vi "Manual_Cam.vi"(4 "Frames in sequence":u32, 6 "Image in":variant, 7 "Camera-specific in":variant, 8 "Save path":path, 9 "Capture mode":enum16{"Single frame", "Sequence"}(ring), 10 "Exposure time (s)":dbl, 11 "Operation":T2(ring)) -> (3 "Status":T1, 5 "Camera-specific out":variant)   [LabVIEW 2015]
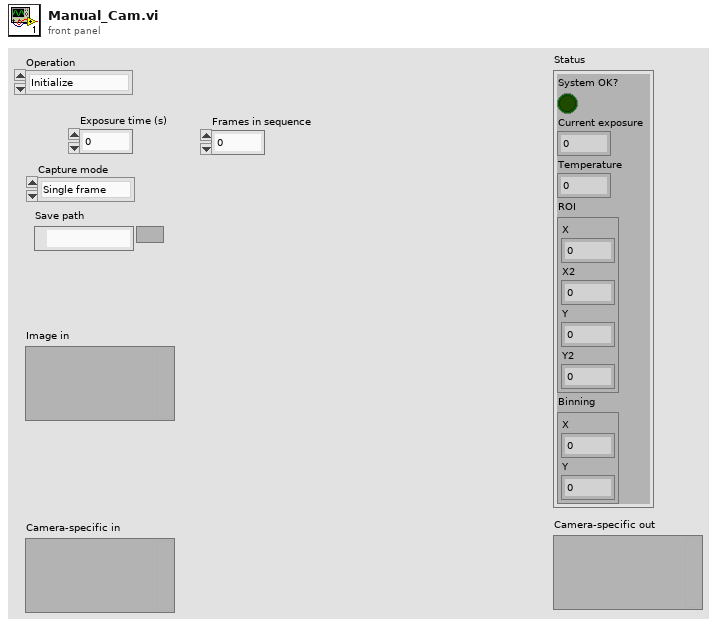
[diagram p1: front panel]
types:
  T1 = cluster{"System OK?":bool, "Current exposure":dbl, "Temperature":dbl, "ROI":cluster{"X":u32, "X2":u32, "Y":u32, "Y2":u32}, "Binning":cluster{"X":u32, "Y":u32}}
  T2 = enum16{"Initialize", "Shut down", "Set capture mode", "Set exposure", "Trigger and read", "Get status", "Other settings"}
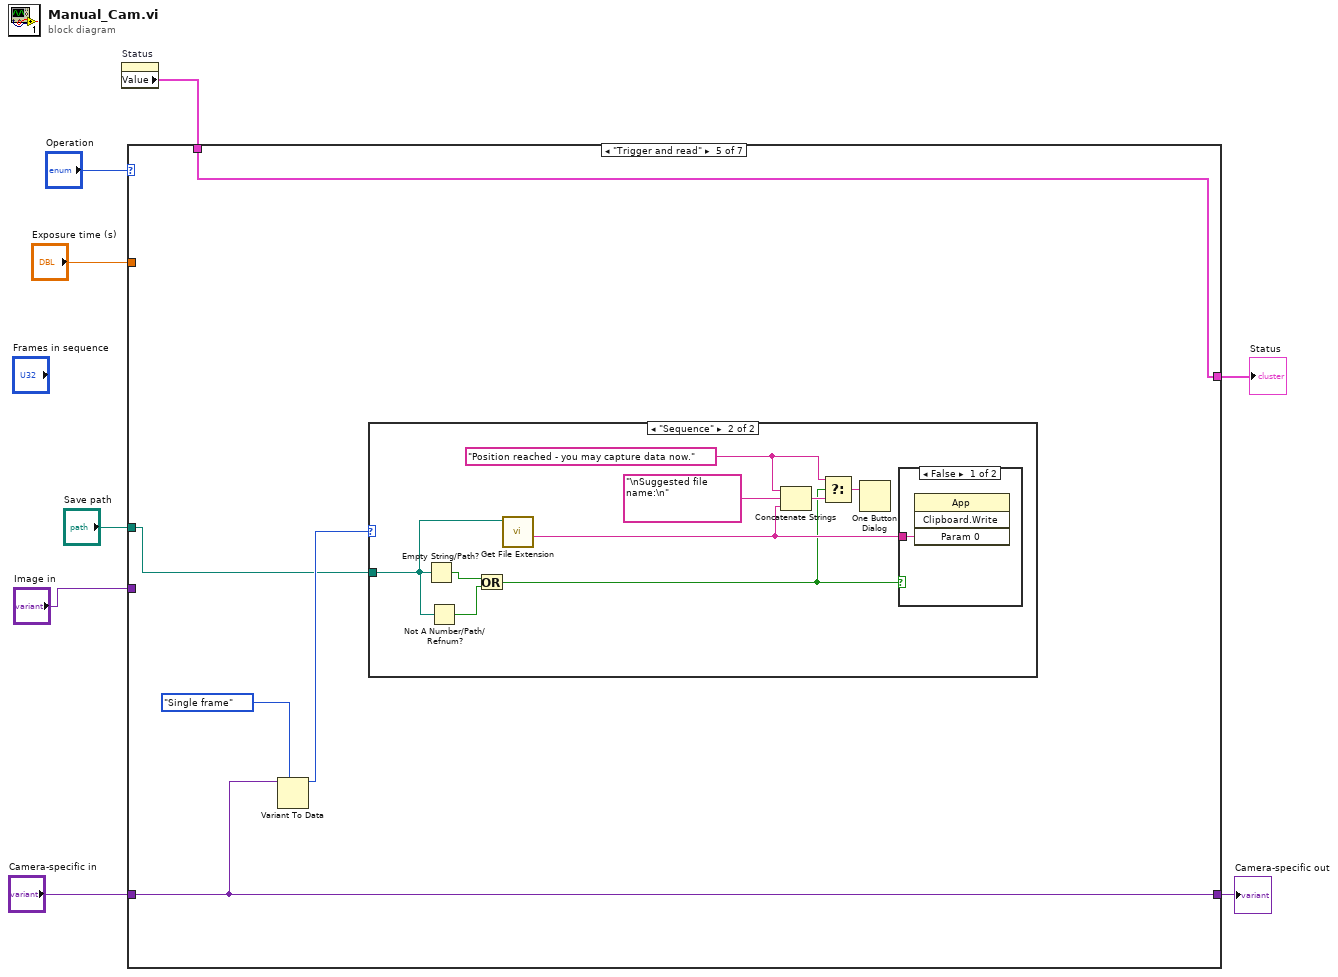
[diagram p0: block diagram]
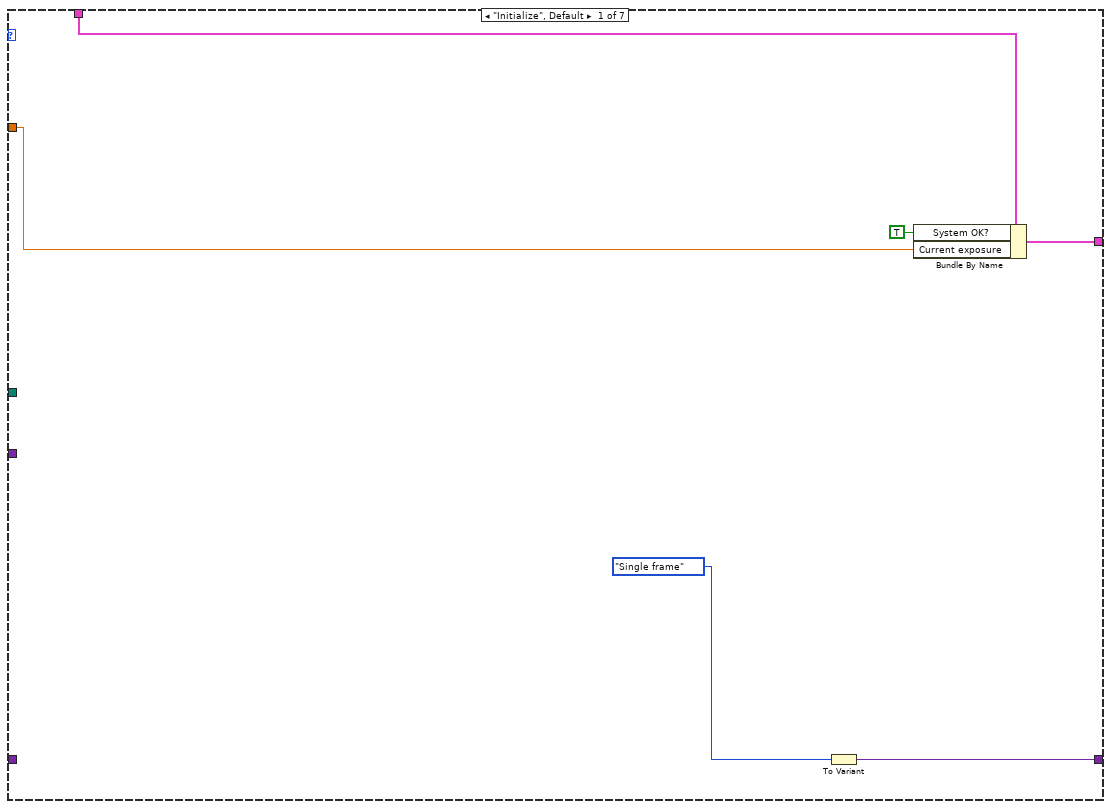
[diagram p2: hidden frame]
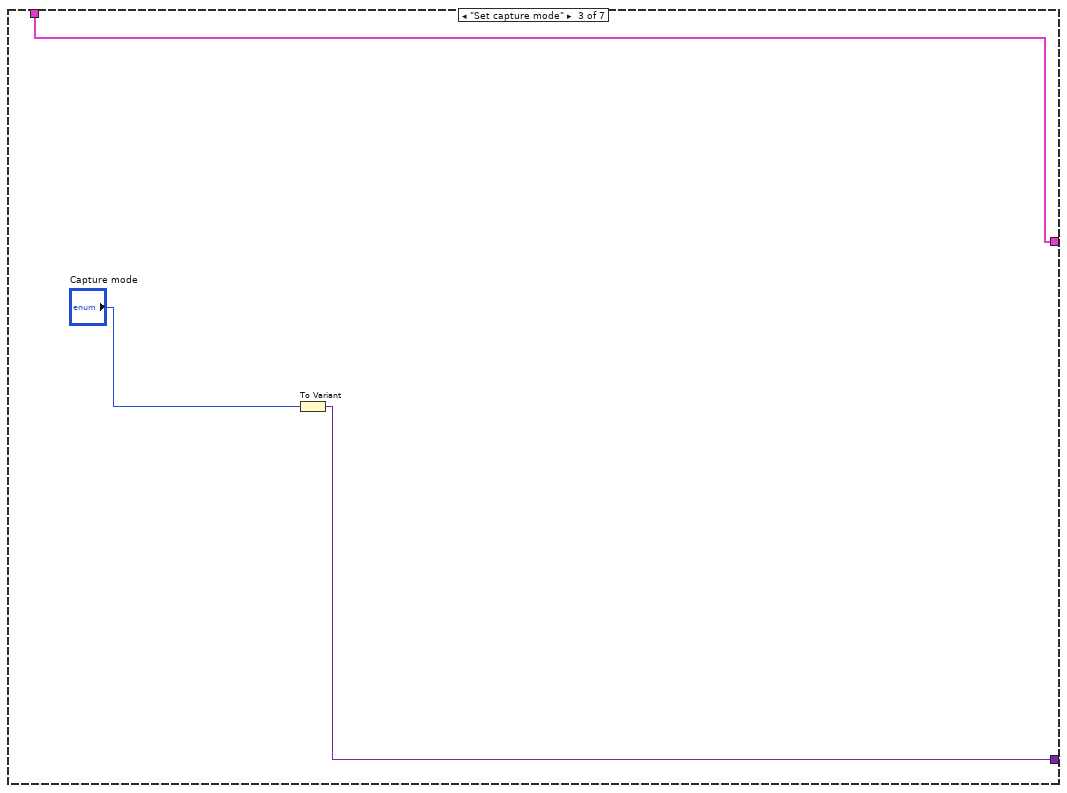
[diagram p4: hidden frame]
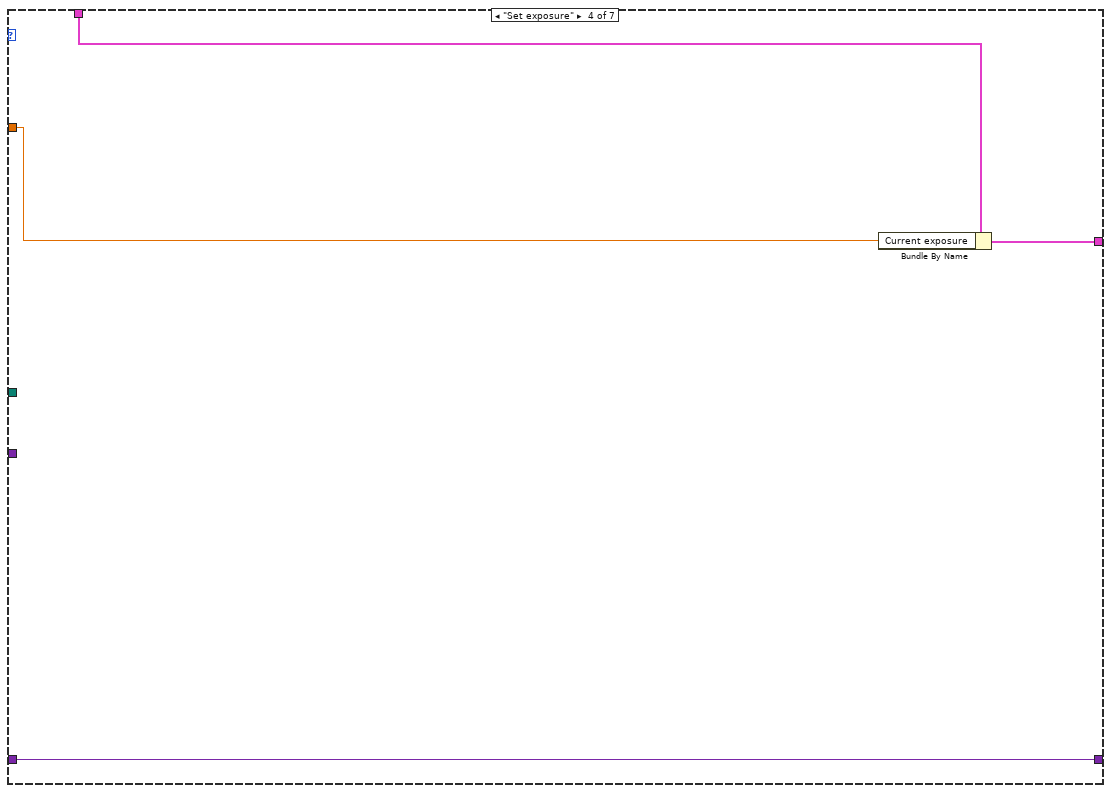
[diagram p5: hidden frame]
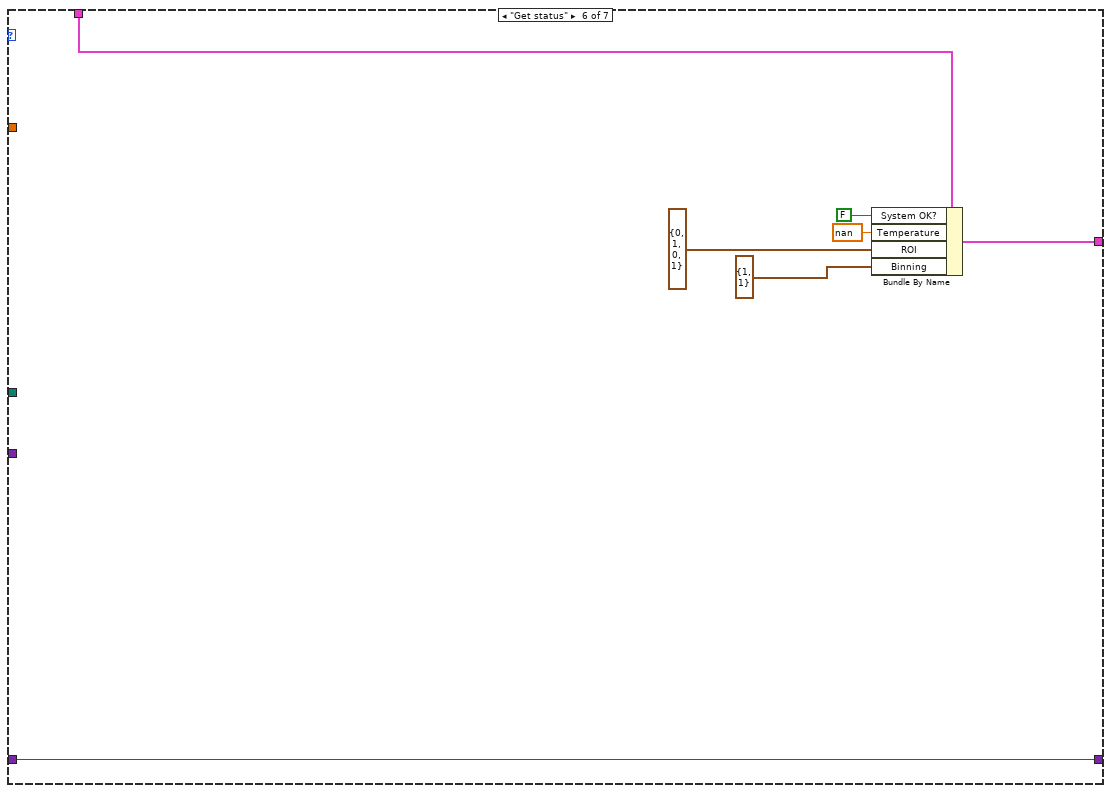
[diagram p8: hidden frame]
diagram:
  n1 = property on="Status" class="Clust (strict)"() -> ("Value"=w6:T1)  [unwired: 2 in, 2 out]
  n2 = case shown="\"Trigger and read\"" "Operation" {
    tunnel: "Exposure time (s)" -> [w12 _ _ w21 _ _ _]
    tunnel: w6 -> [w14 w16 w19 w23 w28 w45 w47]
    tunnel: [w13 w16 w19 w22 w28 w44 w47] -> w5
    tunnel: "Save path" -> [_ _ _ _ w24 _ _]
    tunnel: "Image in" -> [_ _ _ _ _ _ _]
    tunnel: [w10 w15 w17 w20 w27 w39 w46] -> w2
    tunnel: "Camera-specific in" -> [_ w15 _ w20 w27 w39 w46]
    frame "Initialize", Default {
      n3 = To Variant(anything=enum16{"Single frame", "Sequence"}."Single frame" ("Capture mode")) -> (Variant=w10:variant)
      n4 = Bundle By Name(cluster=w14, "System OK?"=TRUE, "Current exposure"=w12) -> (w13:T1)
    }
    frame "Shut down" {
    }
    frame "Set capture mode" {
      n5 = To Variant(anything="Capture mode") -> (Variant=w17:variant)
    }
    frame "Set exposure" {
      n6 = Bundle By Name(cluster=w23, "Current exposure"=w21) -> (w22:T1)
    }
    frame "Trigger and read" {
      n7 = Variant To Data(type=enum16{"Single frame", "Sequence"}."Single frame" ("Capture mode"), Variant=w27) -> (data=w25:enum16{"Single frame", "Sequence"})  [unwired: 1 in, 1 out]
      n8 = case shown="\"Sequence\"" w25 {
        tunnel: w24 -> [_ w31]
        frame "Single frame", Default {
        }
        frame "Sequence" {
          w32 = "Position reached - you may capture data now." ("message")
          n9 = Empty String/Path?(string/path=w31) -> (empty?=w35:bool)
          n10 = Not A Number/Path/Refnum?(number/path/refnum=w31) -> (NaN/Path/Refnum?=w36:bool)
          n11 = Or(x=w35, y=w36) -> (x .or. y?=w29:bool)
          n12 = call <vilib>:"Get File Extension.vi"("file"=w31) -> ("filename without extension"=w30:string)  [unwired: 6 in, 4 out]
          n13 = Concatenate Strings(w32, "\nSuggested file name:\n" ("string"), w30) -> (w33:string)
          n14 = Select(t=w32, s=w29, f=w33) -> (s? t:f=w37:string)
          n15 = One Button Dialog(message=w37) -> ()  [unwired: 1 in, 1 out]
          n16 = case shown="False" w29 {
            tunnel: w30 -> [w38 _]
            frame False {
              n17 = invoke class="App" method="Clipboard.Write"("Param 0"=w38) -> ()  [unwired: 3 in, 4 out]
            }
            frame True {
            }
          }
        }
      }
    }
    frame "Get status" {
      n18 = Bundle By Name(cluster=w45, "System OK?"=FALSE, "Temperature"=nan, "ROI"=cluster{"X":u32, "X2":u32, "Y":u32, "Y2":u32} {"X"=0, "X2"=1, "Y"=0, "Y2"=1}, "Binning"=cluster{"X":u32, "Y":u32} {"X"=1, "Y"=1}) -> (w44:T1)
    }
    frame "Other settings" {
    }
  }
  "Status" <- w5
  "Camera-specific out" <- w2
